vi "Express VI - Scaling and Mapping.vi"() -> ()   [LabVIEW 2023]
doc: "This Example shows how to use the Scaling and Mapping Express VI to scale an input."
panel:
  out "Sound level [db]":dbl(knob) scale=70.0..120.0
  in  "Sound pressure [pa]":dbl(slide)=1.0 scale=0.0..10.0
  in  "Stop":bool
  # "Overview: Demonstrates the use of the Scaling and Mapping Express VI to scale a value.\nRequirements: LabVIEW Full Development System\nInstructions:\n1. Run the VI.\n2. Change the value of the Sound pressure slider.\n3. Click Stop to stop the VI."
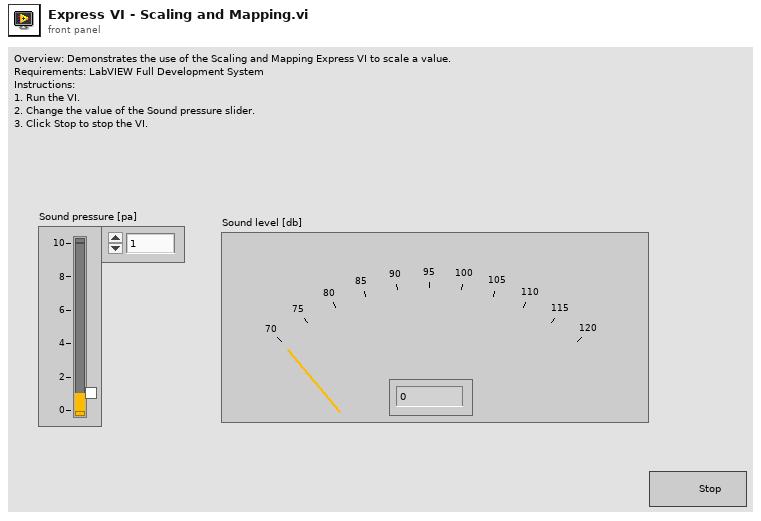
[diagram p1: front panel]
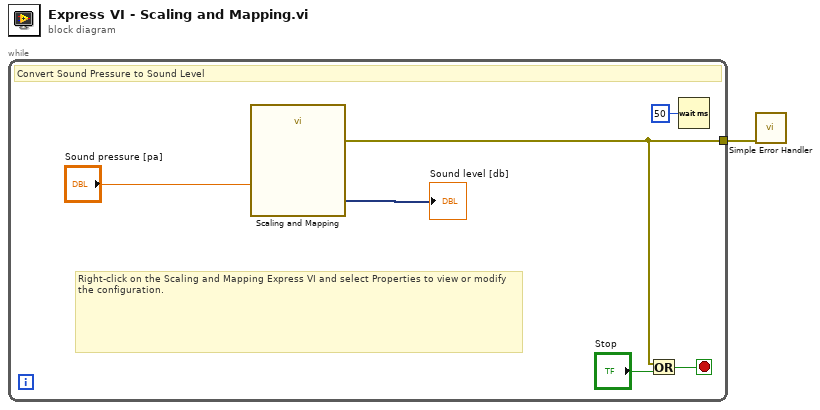
[diagram p0: block diagram]
diagram:
  n1 = while {
    tunnel: [w2] -> w1
    stop <- w3 stop-if-true
    # "Right-click on the Scaling and Mapping Express VI and select Properties to view or modify the configuration."
    # "Convert Sound Pressure to Sound Level"
    n2 = call "Scaling and Mapping"("Signals"="Sound pressure [pa]") -> ("error out"=w2:errorcluster, "Scaled Signals"=→"Sound level [db]":dynamicdata)  [unwired: 9 in]
    n3 = Or(x=w2, y="Stop") -> (x .or. y?=w3:bool)
    n4 = Wait (ms)(milliseconds to wait=u32 50) -> ()  [unwired: 1 out]
  }
  n5 = call <vilib>:"Simple Error Handler.vi"("error in (no error)"=w1) -> ()  [unwired: 4 in, 5 out]
